vi "Step_SetPosition.vi"(6 "Position":dbl, 7 "device_reference":i32, 8 "error in (no error)":errorcluster, 10 "Settings":T1={"device_name"="", "pitch"={"Value"=0.0, "Min"=0.0, "Max"=0.0, "StepSize"=0.0, "Tolerance"=0.0, "ValueActual"=0.0}, "position"={"Value"=0.0, "Min"=0.0, "Max"=0.0, "StepSize"=0.0, "Tolerance"=0.0, "ValueActual"=0.0}, "lowspeed"={"Value"=0.0, "Min"=0.0, "Max"=0.0, "StepSize"=0.0, "Tolerance"=0.0, "ValueActual"=0.0}, "highspeed"={"Value"=0.0, "Min"=0.0, "Max"=0.0, "StepSize"=0.0, "Tolerance"=0.0, "ValueActual"=0.0}, "motor_status"=enum."off", "InitDelay"={"Value"=0.0, "Min"=0.0, "Max"=0.0, "StepSize"=0.0, "Tolerance"=0.0, "ValueActual"=0.0}, "stepsequence"=[], "step"=enum."off", "AutoStep"=enum."off", "MinMonMaxCounts"={"Value"=1000.0, "Min"=0.0, "Max"=0.0, "StepSize"=0.0, "Tolerance"=0.0, "ValueActual"=0.0}, "MinMonMeanCountsRaw"={"Value"=1000.0, "Min"=0.0, "Max"=0.0, "StepSize"=0.0, "Tolerance"=0.0, "ValueActual"=0.0}, "AutoStepTimeout"={"Value"=30000.0, "Min"=0.0, "Max"=0.0, "StepSize"=0.0, "Tolerance"=0.0, "ValueActual"=0.0}}, 11 "WindmillDevice in":refnum<class "WindmillDevice.lvclass">) -> (0 "error out":errorcluster, 3 "WindmillDevice out":refnum<class "WindmillDevice.lvclass">)   [LabVIEW 2020, in "WindmillDevice.lvclass"]
uses:
  WindmillDevice.lvclass
  settingsArcus_TypDef.ctl
  shared/numericVariable_TypeDef.ctl
  WindmillDevice.lvclass/WindmillDevice.ctl
  shared/CompressAndUpdate(Poly)/CompressAndUpdate(Numeric).vi
  BaseDriver/BaseDriver.lvclass
panel:
  out "Settings.AutoStepTimeout.Value":dbl
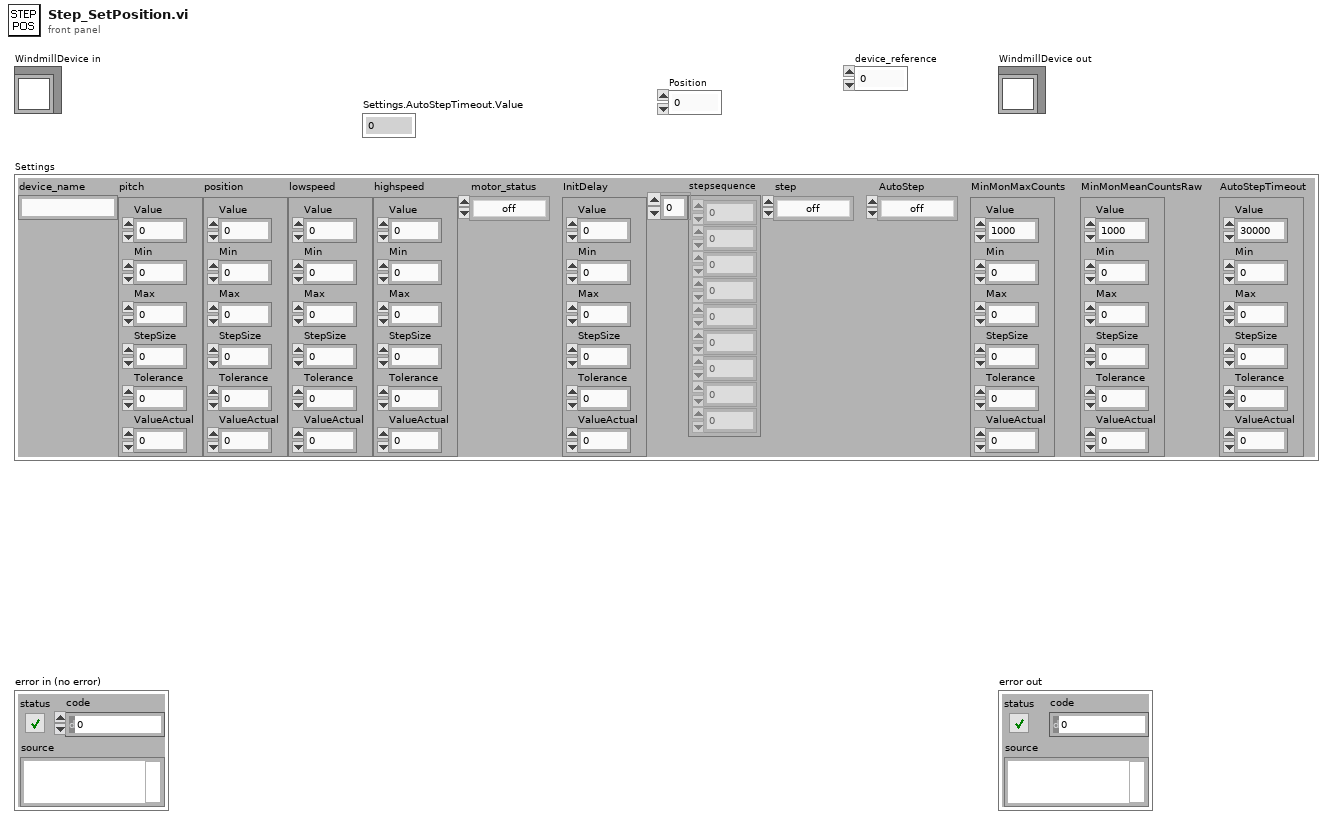
[diagram p1: front panel]
types:
  T1 = typedef "WindmillDevice.lvclass/settingsArcus_TypDef.ctl" = cluster{"device_name":string, "pitch":T2, "position":T2, "lowspeed":T2, "highspeed":T2, "motor_status":enum16{"off", "on"}, "InitDelay":T2, "stepsequence":dbl[], "step":enum16{"off", "on"}, "AutoStep":enum16{"off", "on"}, "MinMonMaxCounts":T2, "MinMonMeanCountsRaw":T2, "AutoStepTimeout":T2}
  T2 = typedef "BaseDriver.lvclass/numericVariable_TypeDef.ctl" = cluster{"Value":dbl, "Min":dbl, "Max":dbl, "StepSize":dbl, "Tolerance":dbl, "ValueActual":dbl}
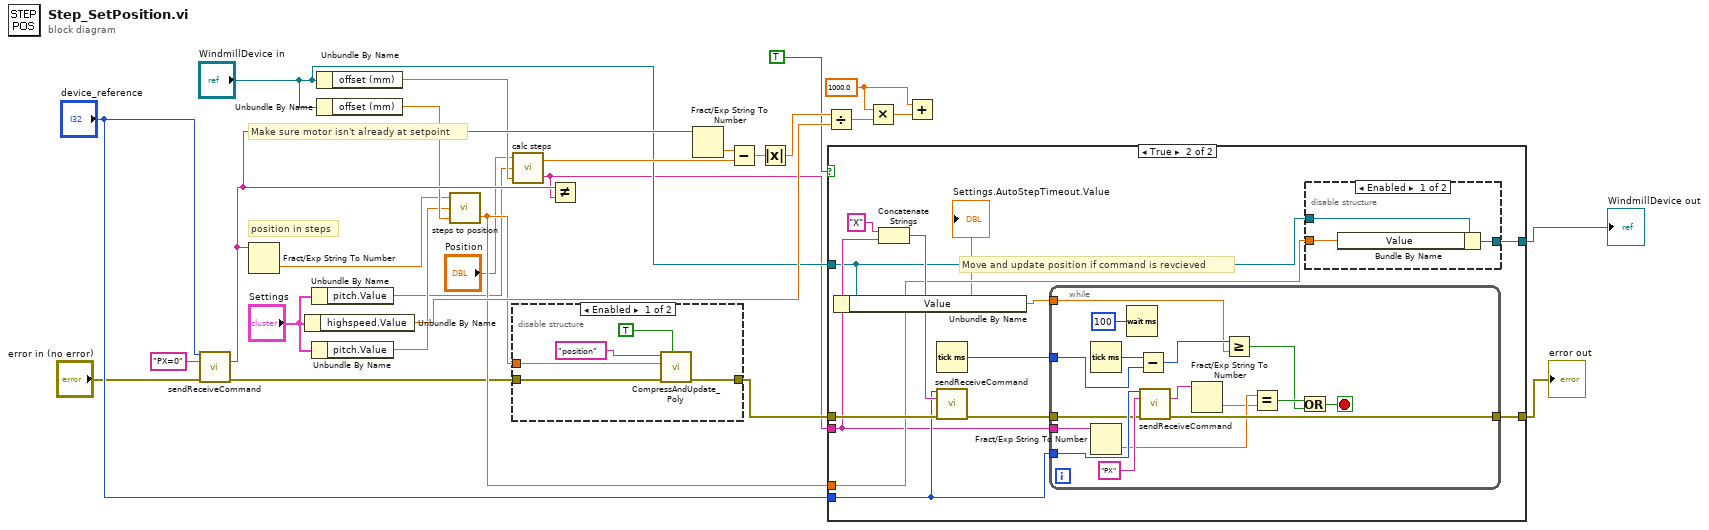
[diagram p0: block diagram]
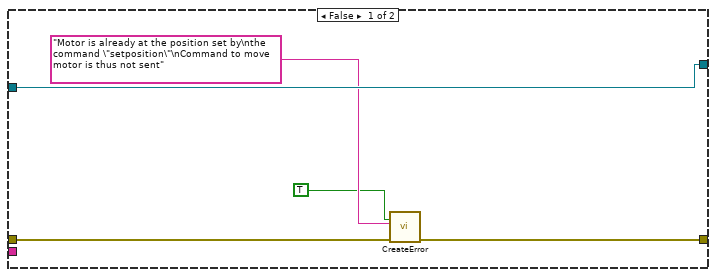
[diagram p3: hidden frame]
diagram:
  w27 = 1000.0 ("x")
  # "position in steps"
  # "Make sure motor isn't already at setpoint"
  n1 = call "sendReceiveCommand.vi"("reference (in)"="device_reference", "write_string"="PX=0", "error in (no error)"="error in (no error)") -> ("read_string"=w19:string, "error out"=w10:errorcluster)  [unwired: 10 in, 1 out]
  n2 = Fract/Exp String To Number(string=w19) -> (number=w13:dbl)  [unwired: 3 in, 1 out]
  n3 = Unbundle By Name("Settings") -> ("highspeed.Value"=w23:dbl)
  n4 = Unbundle By Name("Settings") -> ("pitch.Value"=w8:dbl)
  n5 = Unbundle By Name("Settings") -> ("pitch.Value"=w14:dbl)
  n6 = Unbundle By Name("WindmillDevice in") -> ("offset (mm)"=w9:dbl)
  n7 = Unbundle By Name("WindmillDevice in") -> ("offset (mm)"=w15:dbl)
  n8 = call "steps to position.vi"("Offset (mm)"=w15, "Pitch"=w14, "position (steps)"=w13) -> ("Position  (mm)"=w17:dbl)  [unwired: 1 in]
  n9 = call "calc steps.vi"("Offset (mm)"=w9, "Pitch"=w8, "Position to set (mm)"="Position") -> ("# counts"=w2:string, "pos to set (steps)"=w21:dbl)
  n10 = disable-structure shown="Enabled" {
    disable-tunnel: w10 -> [w31 _]
    disable-tunnel: [w30 _] -> w11
    disable-tunnel: w17 -> [w29 _]
    frame Enabled {
      n11 = call-poly "CompressAndUpdate_Poly.vi"("force CVT update (false)"=TRUE, "error in"=w31, "Numeric"=w29, "command or variable name"="position") -> ("error out"=w30:errorcluster)  [unwired: 7 in]
    }
    frame Disabled {
    }
  }
  n12 = Not Equal?(x=w19, y=w2) -> ()  [unwired: 1 out]
  n13 = Fract/Exp String To Number(string=w19) -> (number=w20:dbl)  [unwired: 3 in, 1 out]
  n14 = Subtract(x=w20, y=w21) -> (x-y=w22:dbl)
  n15 = Absolute Value(x=w22) -> (abs(x)=w26:dbl)
  n16 = Divide(x=w26, y=w23) -> (x/y=w24:dbl)
  n17 = case shown="True" TRUE {
    tunnel: "device_reference" -> [_ w44]
    tunnel: w2 -> [_ w41]
    tunnel: w11 -> [w36 w47]
    tunnel: "WindmillDevice in" -> [w37 w39]
    tunnel: w17 -> [_ w46]
    tunnel: [w35 w42] -> w6
    tunnel: [w37 w45] -> w7
    frame False {
      n18 = call "CreateError.vi"("Warning"=TRUE, "user error in"=w36, "error message (\"\")"="Motor is already at the position set by\nthe command \"setposition\"\nCommand to move motor is thus not sent" ("error message (\"\")")) -> ("user error  out"=w35:errorcluster)  [unwired: 8 in]
    }
    frame True {
      # "Move and update position if command is revcieved"
      n19 = Unbundle By Name(w39) -> ("Value"=w38:dbl)
      "Settings.AutoStepTimeout.Value" <- w38
      n20 = Concatenate Strings("X" ("raw_cmd"), w41) -> (w48:string)
      n21 = Tick Count (ms)() -> (millisecond timer value=w40:u32)
      n22 = call "sendReceiveCommand.vi"("reference (in)"=w44, "write_string"=w48, "error in (no error)"=w47) -> ("error out"=w43:errorcluster)  [unwired: 10 in, 2 out]
      n23 = while {
        tunnel: w44 -> [w64]
        tunnel: w43 -> [w62]
        tunnel: [w61] -> w42
        tunnel: w41 -> [w54]
        tunnel: w40 -> [w57]
        tunnel: w38 -> [w50]
        stop <- w59 stop-if-true
        n24 = Tick Count (ms)() -> (millisecond timer value=w58:u32)
        n25 = Fract/Exp String To Number(string=w54) -> (number=w52:dbl)  [unwired: 3 in, 1 out]
        n26 = Wait (ms)(milliseconds to wait=u32 100) -> ()  [unwired: 1 out]
        n27 = Subtract(x=w58, y=w57) -> (x-y=w56:u32)
        n28 = call "sendReceiveCommand.vi"("reference (in)"=w64, "write_string"="PX", "error in (no error)"=w62) -> ("read_string"=w53:string, "error out"=w61:errorcluster)  [unwired: 10 in, 1 out]
        n29 = Fract/Exp String To Number(string=w53) -> (number=w51:dbl)  [unwired: 3 in, 1 out]
        n30 = Greater Or Equal?(x=w56, y=w50) -> (x >= y?=w55:bool)
        n31 = Equal?(x=w52, y=w51) -> (x = y?=w60:bool)
        n32 = Or(x=w60, y=w55) -> (x .or. y?=w59:bool)
      }
      n33 = disable-structure shown="Enabled" {
        disable-tunnel: w39 -> [w68 w69]
        disable-tunnel: w46 -> [w67 _]
        disable-tunnel: [w66 w69] -> w45
        frame Enabled {
          n34 = Bundle By Name(cluster=w68, "Value"=w67) -> (w66:refnum<class "WindmillDevice.lvclass">)
        }
        frame Disabled {
        }
      }
    }
  }
  "WindmillDevice out" <- w7
  "error out" <- w6
  n35 = Multiply(x=w27, y=w24) -> (x*y=w25:dbl)
  n36 = Add(x=w27, y=w25) -> ()  [unwired: 1 out]
